vi "Correct_Angle.vi"(8 "Keep Tgt Th":dbl=2.1, 9 "Inverse Th":dbl=2.1, 10 "Tgt Angle":dbl=-1.676203185511142, 11 "Src Angle":dbl=1.3522439893550917) -> (3 "Output Angle":dbl=-1.676203185511142)   [LabVIEW 2014]
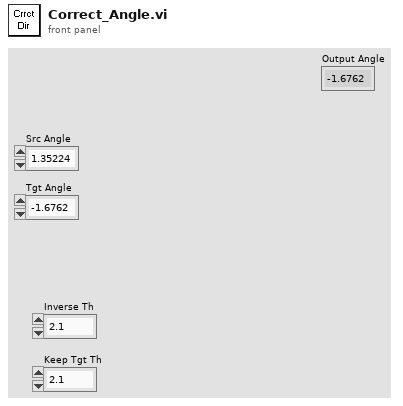
[diagram p1: front panel]
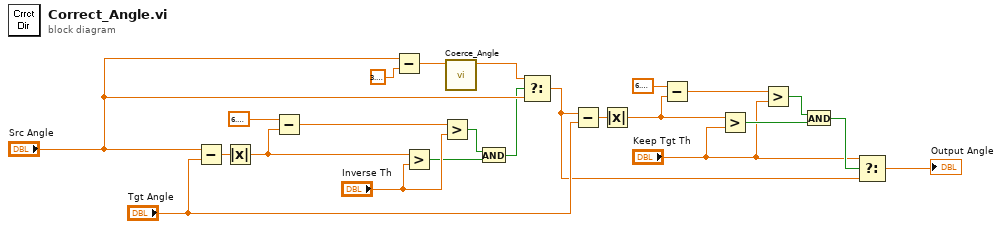
[diagram p0: block diagram]
diagram:
  n1 = Subtract(x="Src Angle", y="Tgt Angle") -> (x-y=w23:dbl)
  n2 = Absolute Value(x=w23) -> (abs(x)=w16:dbl)
  n3 = Subtract(x=6.283185307179586, y=w16) -> (x-y=w15:dbl)
  n4 = Subtract(x="Src Angle", y=3.141592653589793) -> (x-y=w10:dbl)
  n5 = Greater?(x=w16, y="Inverse Th") -> (0:w20:bool)
  n6 = Greater?(x=w15, y="Inverse Th") -> (0:w19:bool)
  n7 = call "Coerce_Angle.vi"("In Angle"=w10) -> ("Out Angle"=w9:dbl)  [unwired: 10 in]
  n8 = And(x=w19, y=w20) -> (x .and. y?=w11:bool)
  n9 = Select(t=w9, s=w11, f="Src Angle") -> (s? t:f=w3:dbl)
  n10 = Subtract(x=w3, y="Tgt Angle") -> (x-y=w8:dbl)
  n11 = Absolute Value(x=w8) -> (abs(x)=w5:dbl)
  n12 = Subtract(x=6.283185307179586, y=w5) -> (x-y=w4:dbl)
  n13 = Greater?(x=w5, y="Keep Tgt Th") -> (0:w18:bool)
  n14 = Greater?(x=w4, y="Keep Tgt Th") -> (0:w17:bool)
  n15 = And(x=w17, y=w18) -> (x .and. y?=w14:bool)
  n16 = Select(t="Keep Tgt Th", s=w14, f=w3) -> (s? t:f=→"Output Angle":dbl)
